vi "hardware_initialize_hardware.vi"(8 "error in (no error)":errorcluster, 11 "lightfield_class in":refnum<class "lightfield_class.lvclass">) -> (0 "error out":errorcluster, 3 "lightfield_class out":refnum<class "lightfield_class.lvclass">)   [LabVIEW 2015, in "lightfield_class.lvclass"]
uses:
  lightfield_class.lvclass
  lightfield_class.lvclass/lightfield_class.ctl
  lightfield-automation-labview/LightField Automation.lvclass
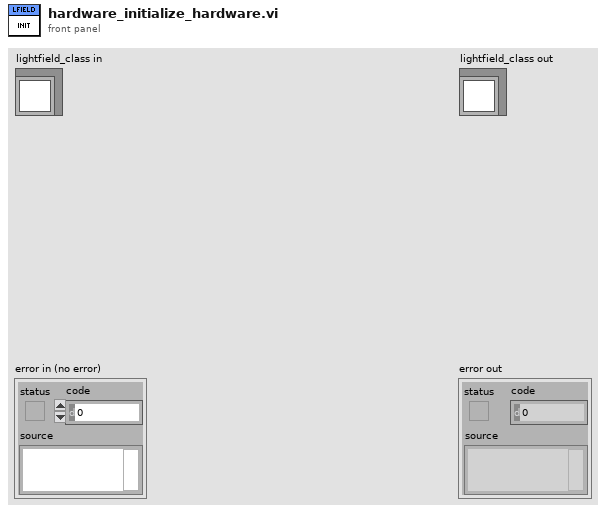
[diagram p1: front panel]
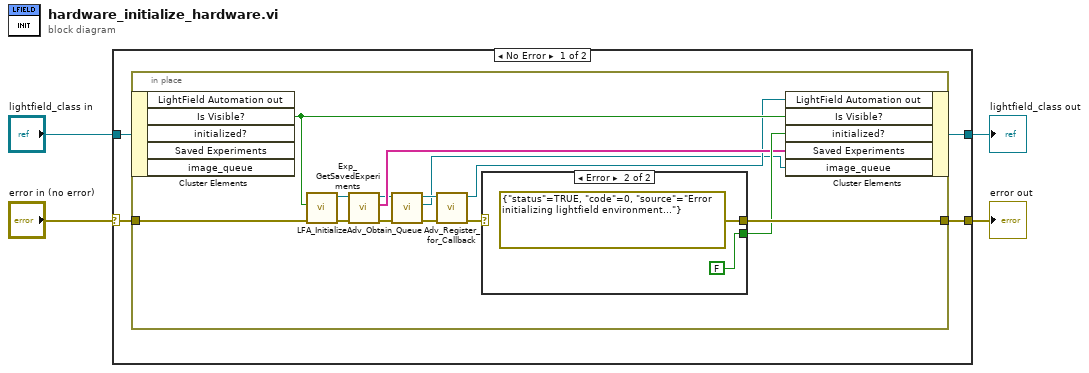
[diagram p0: block diagram]
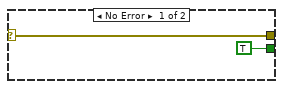
[diagram p2: hidden frame]
diagram:
  n1 = case shown="No Error" "error in (no error)" {
    selector: "error in (no error)" -> [w6 w28]
    tunnel: "lightfield_class in" -> [w8 w27]
    tunnel: [w7 w28] -> w2
    tunnel: [w5 w27] -> w1
    frame No Error {
      n2 = in-place {
        in-place-border: [w18] -> w7
        in-place-border: w6 -> [w21]
        n3 = in-place-cluster #1(w8) -> ("Is Visible?"=w22:bool)  [unwired: 4 out]
        n4 = call "LFA_Initialize.vi"("error in (no error)"=w21, "Is Visible?"=w22) -> ("error out"=w20:errorcluster, "LightField Automation out"=w19:refnum<class "LightField Automation.lvclass">)  [unwired: 8 in]
        n5 = call "Exp_GetSavedExperiments.vi"("error in (no error)"=w20, "LightField Automation in"=w19) -> ("error out"=w15:errorcluster, "Saved Experiments"=w16:string[], "LightField Automation out"=w11:refnum<class "LightField Automation.lvclass">)  [unwired: 7 in]
        n6 = call "Adv_Obtain_Queue.vi"("error in (no error)"=w15, "LightField Automation in"=w11) -> ("error out"=w14:errorcluster, "Queue Reference"=w9:refnum<queue>, "LightField Automation out"=w12:refnum<class "LightField Automation.lvclass">)  [unwired: 7 in]
        n7 = call "Adv_Register_for_Callback.vi"("error in (no error)"=w14, "LightField Automation in"=w12) -> ("error out"=w13:errorcluster, "LightField Automation out"=w10:refnum<class "LightField Automation.lvclass">)  [unwired: 8 in]
        n8 = case shown="Error" w13 {
          selector: w13 -> [w24 _]
          tunnel: [w24 errorcluster {"status"=TRUE, "code"=0, "source"="Error initializing lightfield environment..."} ("error IO")] -> w18
          tunnel: [TRUE FALSE] -> w17
          frame No Error {
          }
          frame Error {
          }
        }
        n9 = in-place-cluster #1("LightField Automation out"=w10, "Is Visible?"=w22, "initialized?"=w17, "Saved Experiments"=w16, "image_queue"=w9) -> (w5:refnum<class "lightfield_class.lvclass">)
      }
    }
    frame Error {
    }
  }
  "error out" <- w2
  "lightfield_class out" <- w1
